vi "Get DVR From Circular Buffer.vi"(7 "Timeout in (ms)":i32=100, 8 "error in (no error)":errorcluster, 10 "Ignore Read Lock":bool, 11 "CIF_NIChn_Fifo_Power_DVR in":refnum<class "CIF_NIChn_Fifo_Power_DVR.lvclass">) -> (0 "error out":errorcluster, 1 "Timeout":bool, 2 "DVRs":refnum<data-value>[](array[refnum]), 3 "CIF_NIChn_Fifo_Power_DVR out":refnum<class "CIF_NIChn_Fifo_Power_DVR.lvclass">, 5 "Remaining timeout (ms)":i32=100)   [LabVIEW 2021, in "CIF_NIChn_Fifo_Power_DVR.lvclass"]
uses:
  CIF_NIChn_Fifo_Power_DVR.lvclass
  ChannelCommon/typedef/Datatype Waveform.ctl
  CIF_NIChn_Fifo_Power_DVR.lvclass/CIF_NIChn_Fifo_Power_DVR.ctl
  ChannelCommon/ChannelCommon.lvlib
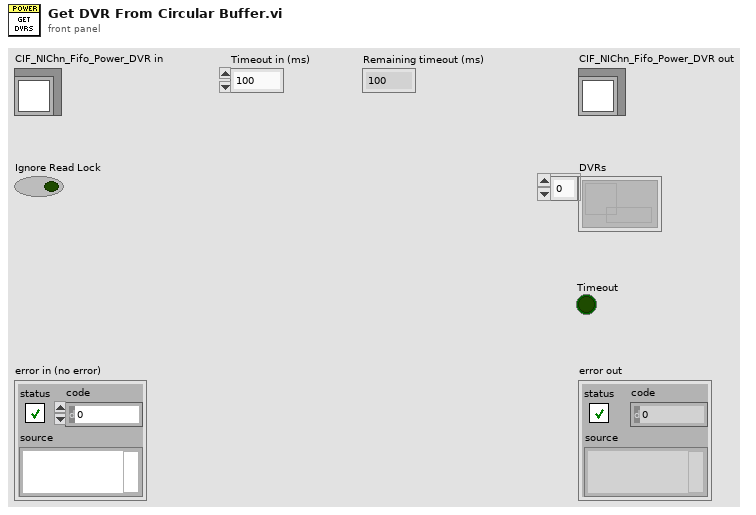
[diagram p1: front panel]
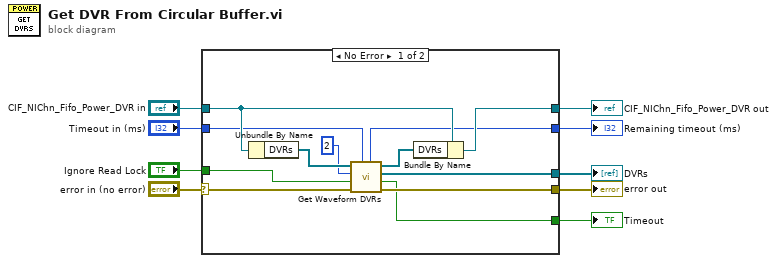
[diagram p0: block diagram]
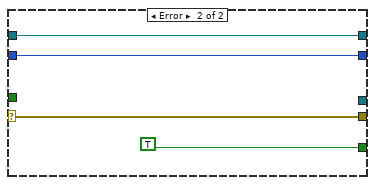
[diagram p2: hidden frame]
diagram:
  n1 = case shown="No Error" "error in (no error)" {
    selector: "error in (no error)" -> [w18 w25]
    tunnel: [w17 w25] -> w8
    tunnel: [w20 w24] -> w6
    tunnel: "CIF_NIChn_Fifo_Power_DVR in" -> [w21 w24]
    tunnel: "Ignore Read Lock" -> [w12 _]
    tunnel: [w15 _] -> w3
    tunnel: [w14 TRUE ("Read Lock")] -> w4
    tunnel: "Timeout in (ms)" -> [w11 w22]
    tunnel: [w10 w22] -> w1
    frame No Error {
      n2 = Unbundle By Name(w21) -> ("DVRs"=w19:refnum<data-value>[])
      n3 = call "Get Waveform DVRs.vi"("Timeout in (ms)"=w11, "error in (no error)"=w18, "Ignore Read Lock"=w12, "Number of Waveforms"=2, "DVR Circular Buffer in"=w19) -> ("error out"=w17:errorcluster, "Timeout"=w14:bool, "DVRs"=w15:refnum<data-value>[], "DVR Circular Buffer out"=w16:refnum<data-value>[], "Remaining timeout (ms)"=w10:i32)  [unwired: 2 in]
      n4 = Bundle By Name(cluster=w21, "DVRs"=w16) -> (w20:refnum<class "CIF_NIChn_Fifo_Power_DVR.lvclass">)
    }
    frame Error {
    }
  }
  "error out" <- w8
  "CIF_NIChn_Fifo_Power_DVR out" <- w6
  "Timeout" <- w4
  "DVRs" <- w3
  "Remaining timeout (ms)" <- w1
